vi "Find Enemies.vi"(11 "Square":refnum<class "Square.lvclass">) -> (2 "Enemy Directions":T1[](array[typedef]))   [LabVIEW 2020, in "SquareBattle.lvlib" / "Square.lvclass"]
doc: "Returns an array of all the directions from this square that contain an enemy. It would be a very good idea to either attack or runaway from enemy squares. Keep in mind that if you and the enemy attack each other, both squares will be eliminated."
uses:
  Square.lvclass
  Direction.ctl
  Square.lvclass/Square.ctl
  SquareBattle.lvlib
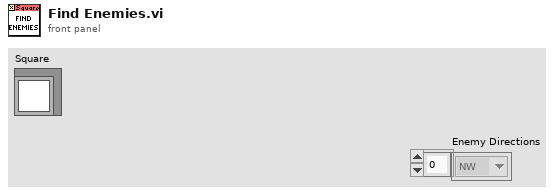
[diagram p1: front panel]
types:
  T1 = typedef "SquareBattle.lvlib/Direction.ctl" = enum16{"NW", "N", "NE", "E", "SE", "S", "SW", "W"}
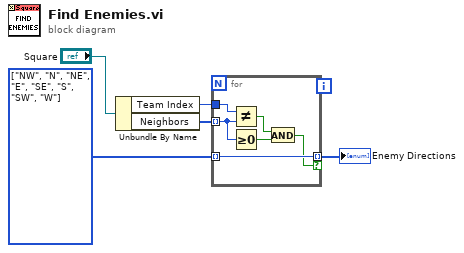
[diagram p0: block diagram]
diagram:
  w2 = T1[] [enum."NW", enum."N", enum."NE", enum."E", enum."SE", enum."S", enum."SW", enum."W"] items=["NW", "N", "NE", "E", "SE", "S", "SW", "W"] ("Enemy Directions")
  n1 = Unbundle By Name("Square") -> ("Team Index"=w4:i32, "Neighbors"=w3:i32[])
  n2 = for {
    tunnel: w4 -> [w10]
    tunnel: w3 -> [w9] mode=indexing
    tunnel: w2 -> [w11] mode=indexing
    tunnel: [w11] -> w1 mode=indexing if=w6
    n3 = Not Equal?(x=w10, y=w9) -> (x != y?=w7:bool)
    n4 = Greater Or Equal To 0?(x=w9) -> (x >= 0?=w8:bool)
    n5 = And(x=w7, y=w8) -> (x .and. y?=w6:bool)
  }
  "Enemy Directions" <- w1
